vi "createNewWorksheet.vi"(8 "error in (no error)":errorcluster, 10 "Worksheet Name":string, 11 "workbook in":refnum<class "workbook.lvclass">) -> (0 "error out":errorcluster, 3 "workbook out":refnum<class "workbook.lvclass">)   [LabVIEW 2017, in "Excel_Specific.lvlib" / "workbook.lvclass"]
uses:
  workbook.lvclass
  workbook.lvclass/workbook.ctl
  worksheet/worksheet.lvclass
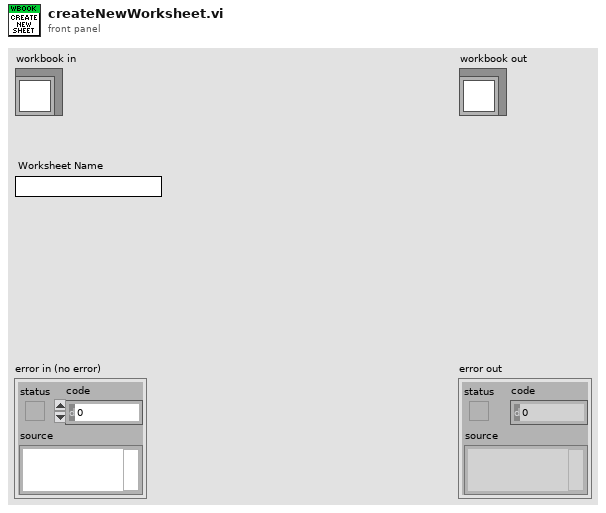
[diagram p1: front panel]
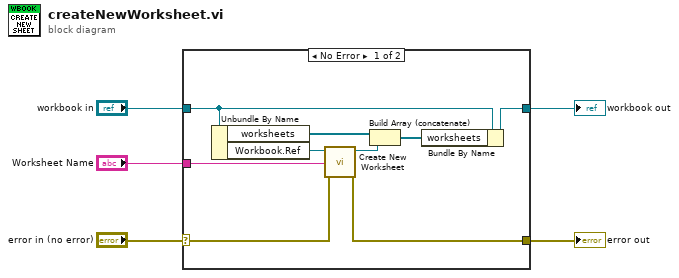
[diagram p0: block diagram]
diagram:
  n1 = case shown="No Error" "error in (no error)" {
    selector: "error in (no error)" -> [w11 w16]
    tunnel: [w6 w16] -> w4
    tunnel: [w10 w15] -> w2
    tunnel: "workbook in" -> [w14 w15]
    tunnel: "Worksheet Name" -> [w12 _]
    frame No Error {
      n2 = Unbundle By Name(w14) -> ("worksheets"=w9:refnum<class "worksheet.lvclass">[], "Workbook.Ref"=w13:refnum<k24>)
      n3 = call "Create New Worksheet.vi"("error in (no error)"=w11, "sheetname"=w12, "Workbook"=w13) -> ("error out"=w6:errorcluster, "worksheet out"=w7:refnum<class "worksheet.lvclass">)  [unwired: 7 in]
      n4 = Build Array (concatenate)(w9, w7) -> (w8:refnum<class "worksheet.lvclass">[])
      n5 = Bundle By Name(cluster=w14, "worksheets"=w8) -> (w10:refnum<class "workbook.lvclass">)
    }
    frame Error {
    }
  }
  "error out" <- w4
  "workbook out" <- w2
